vi "SR SIM921 Get Curve Data.vi"(4 "error in (no error)":errorcluster, 5 "Curve #":i32, 6 "Mainframe slot":u32=3, 7 "VISA session":refnum<visa-resource-name>) -> (0 "error out":errorcluster, 1 "Resistance":dbl[](array[numeric]) format="%.3e", 2 "Temperature":dbl[](array[numeric]) format="%.3e", 3 "dup VISA session":refnum<visa-resource-name>)   [LabVIEW 2019]
doc: "This VI will download and graph a calibration curve from a LakeShore Model 370 AC Resistance Bridge.\nScott Hannahs, <sth@magnet.fsu.edu> NHMFL-FSU, May 2003"
panel:
  out "# of Points":i32
  out "XY Graph":cluster{dbl[], dbl[]}(graph)
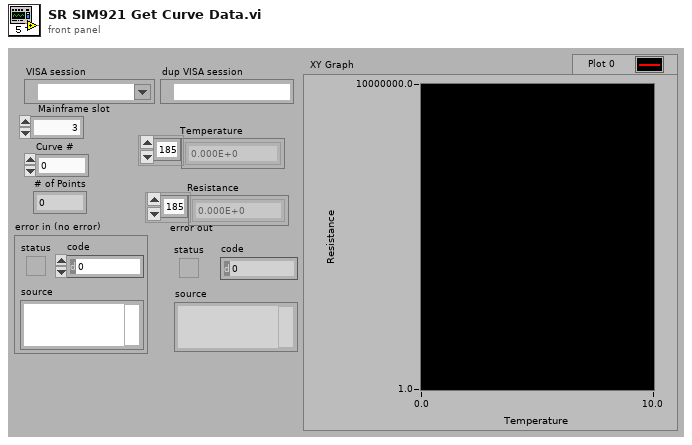
[diagram p1: front panel]
types:
  T1 = cluster{"Curve ID":string, "Serial Number":string, "Data Format":string, "Number of Points":u32}
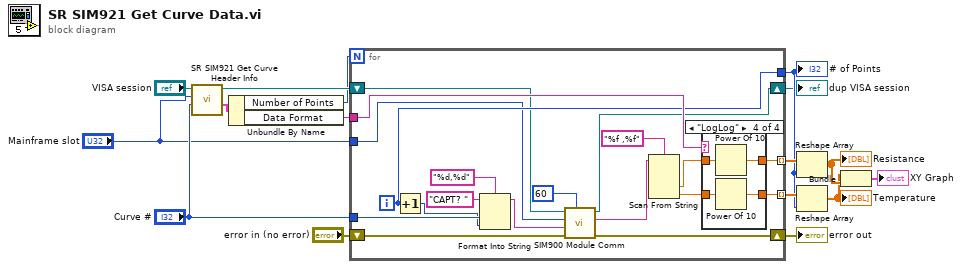
[diagram p0: block diagram]
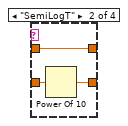
[diagram p3: hidden frame]
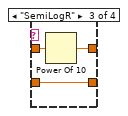
[diagram p4: hidden frame]
diagram:
  n1 = call "SR SIM921 Get Curve Header Info.vi"("Curve #"="Curve #", "SIM Slot #"="Mainframe slot", "VISA session"="VISA session") -> ("Curve Header"=w11:T1, "dup VISA session"=w14:refnum<visa-resource-name>)  [unwired: 2 in, 1 out]
  n2 = Unbundle By Name(w11) -> ("Number of Points"=w4:u32, "Data Format"=w2:string)
  n3 = for {
    N: w4 -> [_]
    tunnel: [w27] -> w16 mode=indexing
    tunnel: [w21] -> w15 mode=indexing
    tunnel: "Curve #" -> [w30]
    tunnel: w2 -> [w29]
    tunnel: [w25] -> w10
    tunnel: "Mainframe slot" -> [w20]
    shift-right: [w18] -> w3
    shift-left: "error in (no error)" -> [w19]
    shift-right: [w23] -> w6
    shift-left: w14 -> [w24]
    i -> [w25]
    n4 = Increment(x=w25) -> (x+1=w26:i32)
    n5 = Format Into String(format string="%d,%d", initial string="CAPT? " ("String to Write"), w30, w26) -> (resulting string=w34:string)  [unwired: 1 in, 1 out]
    n6 = call "SIM900 Module Comm.vi"("Wait (ms)"=u32 60, "Error In"=w19, "Query"=w34, "Slot"=w20, "VISA Resource Name"=w24) -> ("Error Out"=w18:errorcluster, "Response"=w31:string, "dup VISA Session"=w23:refnum<visa-resource-name>)  [unwired: 4 in]
    n7 = Scan From String(format string="%f ,%f", input string=w31) -> (output 1=w28:dbl, output 2=w22:dbl)  [unwired: 4 in, 3 out]
    n8 = case shown="\"LogLog\"" w29 {
      tunnel: w28 -> [w37 w38 w43 w47]
      tunnel: [w37 w38 w42 w46] -> w27
      tunnel: w22 -> [w36 w40 w41 w45]
      tunnel: [w36 w39 w41 w44] -> w21
      frame "Linear", Default {
      }
      frame "SemiLogT" {
        n9 = Power Of 10(x=w40) -> (10^x=w39:dbl)
      }
      frame "SemiLogR" {
        n10 = Power Of 10(x=w43) -> (10^x=w42:dbl)
      }
      frame "LogLog" {
        n11 = Power Of 10(x=w47) -> (10^x=w46:dbl)
        n12 = Power Of 10(x=w45) -> (10^x=w44:dbl)
      }
    }
  }
  "dup VISA session" <- w6
  "# of Points" <- w10
  "error out" <- w3
  n13 = Reshape Array(w16, w10) -> (w8:dbl[])
  "Resistance" <- w8
  n14 = Reshape Array(w15, w10) -> (w7:dbl[])
  "Temperature" <- w7
  n15 = Bundle(w7, w8) -> (→"XY Graph":cluster{dbl[], dbl[]})  [unwired: 1 in]
